vi "Perform Action.vi"(8 "error in (no error)":errorcluster, 10 "Input":variant, 11 "Virt Instrs DIO.lvlib:Virt PWM Generator.lvclass":refnum<class "Virt DAQmx PWM Generator.lvclass">) -> (0 "error out":errorcluster, 2 "Output":variant, 3 "Virt Instrs DIO.lvlib:Virt PWM Generator.lvclass out":refnum<class "Virt DAQmx PWM Generator.lvclass">)   [LabVIEW 2023, in "Virt Instrs DIO.lvlib" / "Virt DAQmx PWM Generator.lvclass"]
uses:
  Virt DAQmx PWM Generator.lvclass
  Virt DAQmx PWM Generator.lvclass/Virt DAQmx PWM Generator.ctl
  Virt Instr Host/Virt Instr Host.lvclass
  Instrument/Instrument.lvclass
  D:/git/HAL/HAL GOOP4/Virt Instr Host/Virt Instr Host.lvclass
  D:/git/HAL/HAL GOOP4/Virt Instr Base/Virt Instr Base.lvclass
  D:/git/HAL/HAL GOOP4/DIO/Virtual DIO/Virt PWM Generator/Virt DAQmx PWM Generator.lvclass
  Virt Instr Base/Virt Instr Base.lvclass
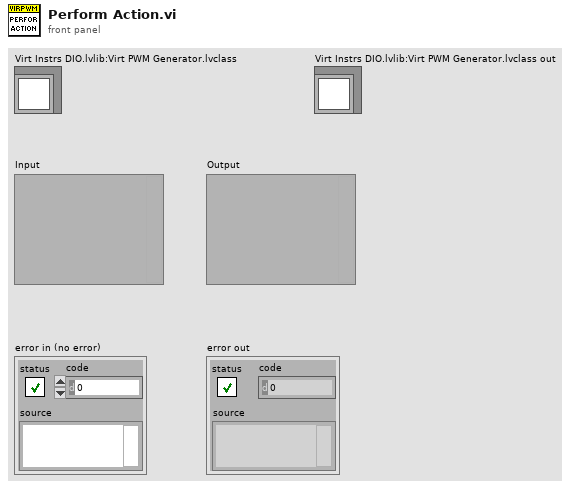
[diagram p1: front panel]
types:
  T1 = cluster{"Channel":string, "PWM Pams":cluster{"Frequency":dbl, "Duty Cycle":dbl}}
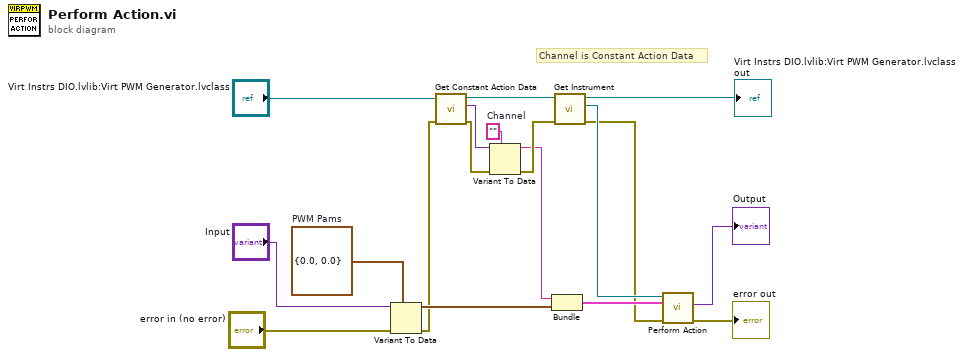
[diagram p0: block diagram]
diagram:
  w1 = cluster{"Frequency":dbl, "Duty Cycle":dbl} {"Frequency"=0.0, "Duty Cycle"=0.0}  # PWM Pams
  w14 = ""  # Channel
  # "Channel is Constant Action Data"
  n1 = Variant To Data(error in="error in (no error)", type=w1, Variant="Input") -> (data=w18:cluster{"Frequency":dbl, "Duty Cycle":dbl}, error out=w16:errorcluster)
  n2 = call "Get Constant Action Data.vi"("error in (no error)"=w16, "Virt Instr Base in"="Virt Instrs DIO.lvlib:Virt PWM Generator.lvclass") -> ("error out"=w17:errorcluster, "Constant Action Data"=w7:variant, "Virt Instr Base out"=w9:refnum<class "Virt DAQmx PWM Generator.lvclass">)  [unwired: 7 in]
  n3 = Variant To Data(error in=w17, type=w14, Variant=w7) -> (data=w13:string, error out=w15:errorcluster)
  n4 = Bundle("Channel"=w13, "PWM Pams"=w18) -> (w6:T1)  [unwired: 1 in]
  n5 = call "Get Instrument.vi"("error in (no error)"=w15, "Virt Instr Base in"=w9) -> ("error out"=w4:errorcluster, "HAL GOOP4.lvlib:Instrument"=w5:refnum<class "Instrument.lvclass">, "Virt Instr Base in"=→"Virt Instrs DIO.lvlib:Virt PWM Generator.lvclass out":refnum<class "Virt DAQmx PWM Generator.lvclass">)  [unwired: 7 in]
  n6 = call "Perform Action.vi"("Error In"=w4, "Input"=w6, "reference in"=w5) -> ("Error Out"=→"error out":errorcluster, "Output"=→"Output":variant)  [unwired: 6 in, 1 out]
